vi "Simulation Record Read.vi"(8 "Error In":errorcluster, 11 "record file":path=path "simulation trace.xml") -> (0 "Error Out":errorcluster, 3 "simulation record":T1={"configuration"={"maxTime"=5.0, "enableVisualization"=TRUE, "Environment Definition"=path "iRobot Navigation State Machine.vi", "Record Location"=path "Simulated iRobot.xml", "autograde?"=TRUE, "interactive?"=FALSE, "Feedback Mode"=enum."debug navigation", "Robot State Charts"=[path "C:/Users/blueuser/Desktop/Robo Sim Berkley/cpsgrader-release-0.4/Simulators/EECS149lab/src/LabVIEW/statechart/Simulation Statechart.vi"], "statechart"=path "iRobot Navigation State Machine.vi"}, "trace"=[], "environment MD5"="", "statechart MD5"="", "record timestamp"=""} {"trace"."sensors"."accelerometer"."z axis (g)" format="%.3f"; "trace"."sensors"."accelerometer"."y axis (g)" format="%.3f"; "trace"."sensors"."accelerometer"."x axis (g)" format="%.3f"})   [LabVIEW 2014]
uses:
  Simulation Record.ctl
  CyberSim interface/Simulation Configuration.ctl
  autograder/feedbackMode.ctl
  Simulation Trace Element.ctl
  shared/Sensors.ctl
  shared/Accelerometer.ctl
  Kobuki/KobukiSensors.ctl
  Kobuki/Kobuki Bumps and WheelDrops.ctl
  Kobuki/Kobuki Buttons.ctl
  Kobuki/Charging Sources Available.ctl
  Simulated Position.ctl
  Simulated Orientation.ctl
  <vilib>/Utility/xml.llb/Read From XML File(string).vi
panel:
  # "Electrical: charging, battery, OI mode"
  # "Sensors: bump, cliff, button, wheel drop, wall, virtual wall"
  # "Motors:"
  # "Song"
  # "Inertia"
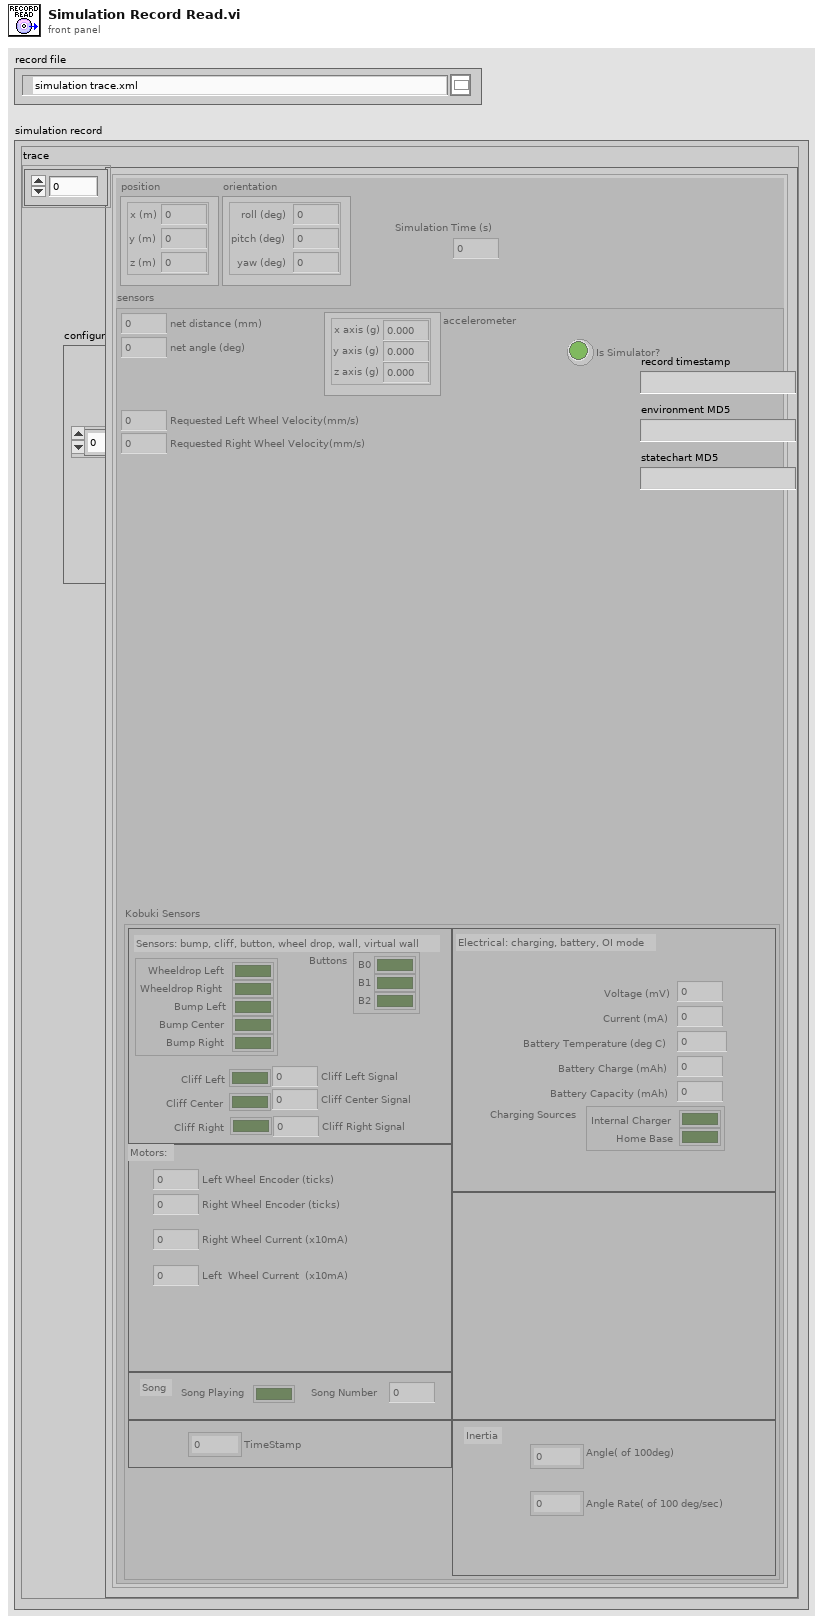
[diagram p1: front panel]
types:
  T1 = typedef "Simulation Record.ctl" = cluster{"configuration":T2, "trace":T4[], "environment MD5":string, "statechart MD5":string, "record timestamp":string}
  T2 = typedef "Simulation Configuration.ctl" = cluster{"maxTime":sgl, "enableVisualization":bool, "Environment Definition":path, "Record Location":path, "autograde?":bool, "interactive?":bool, "Feedback Mode":T3, "Robot State Charts":path[], "statechart":path}
  T3 = typedef "feedbackMode.ctl" = enum32{"debug navigation", "debug hill climb", "autograde navigation", "autograde hill climb"}
  T4 = typedef "Simulation Trace Element.ctl" = cluster{"sensors":T5, "position":T11, "orientation":T12, "Simulation Time (s)":sgl}
  T5 = typedef "Sensors.ctl" = cluster{"net distance (mm)":i32, "net angle (deg)":i32, "accelerometer":T6, "Is Simulator?":bool, "Kobuki Sensors":T7, "Requested Left Wheel Velocity(mm/s)":i32, "Requested Right Wheel Velocity(mm/s)":i32}
  T6 = typedef "Accelerometer.ctl" = cluster{"x axis (g)":dbl, "y axis (g)":dbl, "z axis (g)":dbl}
  T7 = typedef "KobukiSensors.ctl" = cluster{"Bumps + Wheel Drops":T8, "Cliff Left":bool, "Cliff Center":bool, "Cliff Right":bool, "Cliff Left Signal":u16, "Cliff Center Signal":u16, "Cliff Right Signal":u16, "Buttons":T9, "Left Wheel Encoder (ticks)":u16, "Right Wheel Encoder (ticks) ":u16, "Right Wheel Current (x10mA)":i16, "Left  Wheel Current  (x10mA)":i16, "TimeStamp":u16, "Song Playing":bool, "Song Number":u8, "Voltage (mV)":i16, "Current (mA)":i16, "Battery Temperature (deg C)":i16, "Battery Charge (mAh)":i16, "Battery Capacity (mAh)":i16, "Charging Sources":T10, "Angle( of 100deg)":i16, "Angle Rate( of 100 deg/sec)":i16}
  T8 = typedef "Kobuki Bumps and WheelDrops.ctl" = cluster{"Wheeldrop Left":bool, "Wheeldrop Right":bool, "Bump Left":bool, "Bump Center":bool, "Bump Right":bool}
  T9 = typedef "Kobuki Buttons.ctl" = cluster{"B0":bool, "B1":bool, "B2":bool}
  T10 = typedef "Charging Sources Available.ctl" = cluster{"Internal Charger":bool, "Home Base":bool}
  T11 = typedef "Simulated Position.ctl" = cluster{"x (m)":sgl, "y (m)":sgl, "z (m)":sgl}
  T12 = typedef "Simulated Orientation.ctl" = cluster{"roll (deg)":sgl, "pitch (deg)":sgl, "yaw (deg)":sgl}
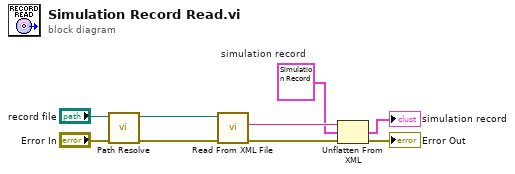
[diagram p0: block diagram]
diagram:
  w3 = T1 {"configuration"={"maxTime"=0.0, "enableVisualization"=FALSE, "Environment Definition"=path "", "Record Location"=path "", "autograde?"=FALSE, "interactive?"=FALSE, "Feedback Mode"=enum."debug navigation", "Robot State Charts"=[path "C:/Users/blueuser/Desktop/Robo Sim Berkley/cpsgrader-release-0.4/Simulators/EECS149lab/src/LabVIEW/statechart/Simulation Statechart.vi"], "statechart"=path ""}, "trace"=[], "environment MD5"="", "statechart MD5"="", "record timestamp"=""}  # simulation record
  n1 = call "Path Resolve.vi"("Error In"="Error In", "absolute or relative path"="record file") -> ("Error Out"=w7:errorcluster, "resolved path"=w8:path)  [unwired: 8 in]
  n2 = call-poly <vilib>:"Read From XML File.vi"("error in (no error)"=w7, "XML File Path"=w8) -> ("error out"=w5:errorcluster, "XML Elements"=w4:string)  [unwired: 7 in, 1 out]
  n3 = Unflatten From XML(xml string=w4, type=w3, error in (no error)=w5) -> (value=→"simulation record":T1, error out=→"Error Out":errorcluster)
